vi "Init.vi"(8 "error in (no error)":errorcluster, 11 "WebSocket Manager in":refnum<class "WebSocket Manager.lvclass">) -> (0 "error out":errorcluster, 3 "WebSocket Manager out":refnum<class "WebSocket Manager.lvclass">)   [LabVIEW 2020, in "HTTP Server.lvlib" / "WebSocket Manager.lvclass"]
uses:
  WebSocket Manager.lvclass
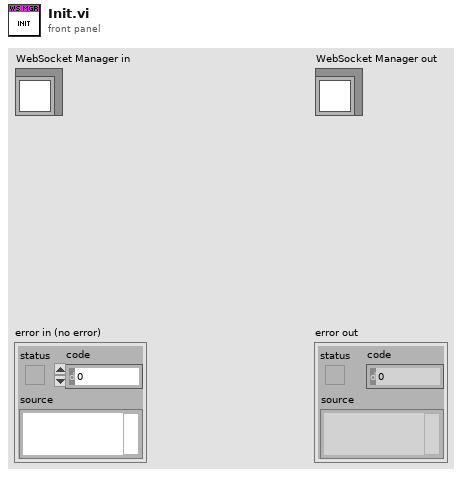
[diagram p1: front panel]
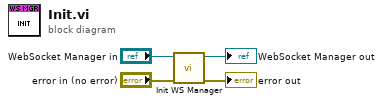
[diagram p0: block diagram]
diagram:
  n1 = call-dynamic "Init WS Manager.vi"("error in (no error)"="error in (no error)", "WebSocket Manager in"="WebSocket Manager in") -> ("error out"=→"error out":errorcluster, "WebSocket Manager out"=→"WebSocket Manager out":refnum<class "WebSocket Manager.lvclass">)  [unwired: 8 in]
